vi "ST_do_SQL_transaction.vi"(6 "station":T1, 8 "error_in":errorcluster, 10 "SQL_transaction":string[](array[string]), 11 "SQL_connection_reference":T2) -> (0 "error_out":errorcluster)   [LabVIEW 2020]
uses:
  <vilib>/addons/database/Connection.llb/Conn ObjectReference.ctl
  station.ctl
  <vilib>/addons/database/Auxilliary.llb/DB Tools Transaction.ctl
  FGV/DIAGNOSTICS_message_history_buffer/FGV_PROXY_DIAGNOSTICS_message_history_buffer.ctl
  <vilib>/addons/database/Connection.llb/Conn Transaction.vi
  <vilib>/addons/database/Connection.llb/Conn Execute.vi
  <vilib>/addons/database/Recordset.llb/Rec Destroy - Connection.vi
  <vilib>/addons/database/NI_Database_API.lvlib
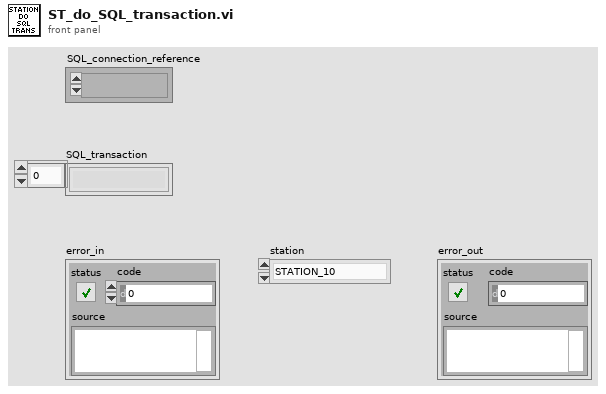
[diagram p1: front panel]
types:
  T1 = typedef "station.ctl" = enum16{"STATION_10", "STATION_20", "STATION_30", "STATION_40", "STATION_50", "STATION_60", "STATION_70", "STATION_80", "STATION_90", "STATION_100", "STATION_110", "STATION_120", "STATION_165", "MAIN"}
  T2 = typedef "NI_Database_API.lvlib/Conn ObjectReference.ctl" = refnum<k1>
  T3 = typedef "FGV_PROXY_DIAGNOSTICS_message_history_buffer.ctl" = enum16{"initialize", "add_TCP_PLC_to_PC", "add_TCP_PC_to_PLC", "add_SQL_PC_to_DB", "add_SQL_transaction", "add_SQL_DB_to_PC", "get_station", "get_all", "clear_station", "clear_all", "save_log"}
  T4 = typedef "NI_Database_API.lvlib/DB Tools Transaction.ctl" = enum16{"begin", "commit", "rollback"}
  T5 = typedef "NI_Database_API.lvlib/Rec ObjectReference.ctl" = refnum<k1>
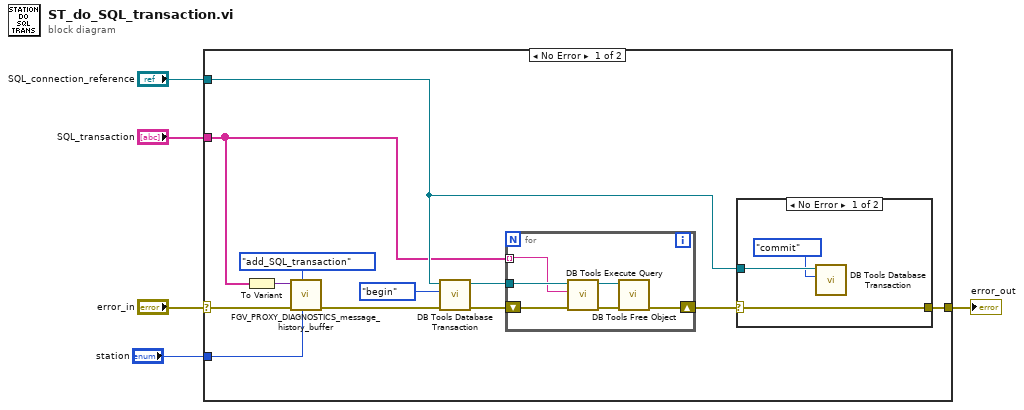
[diagram p0: block diagram]
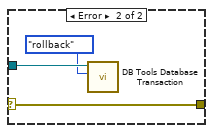
[diagram p2: hidden frame]
diagram:
  n1 = case shown="No Error" "error_in" {
    selector: "error_in" -> [w9 w30]
    tunnel: [w13 w30] -> w5
    tunnel: "SQL_transaction" -> [w7 _]
    tunnel: "SQL_connection_reference" -> [w12 _]
    tunnel: "station" -> [w6 _]
    frame No Error {
      n2 = To Variant(anything=w7) -> (Variant=w11:variant)
      n3 = call "FGV_PROXY_DIAGNOSTICS_message_history_buffer.vi"("station"=w6, "options"=FGV_PROXY_DIAGNOSTICS_message_history_buffer."add_SQL_transaction", "error_in"=w9, "input"=w11) -> ("error_out"=w8:errorcluster)  [unwired: 6 in, 1 out]
      n4 = call-poly <vilib>:"DB Tools Database Transaction.vi"("error in (no error)"=w8, "operation (begin)"=DB_Tools_Transaction."begin", "connection reference"=w12) -> ("error out"=w16:errorcluster, "connection reference out"=w15:T2)  [unwired: 3 in]
      n5 = for {
        tunnel: w15 -> [w20]
        shift-right: [w19] -> w14
        shift-left: w16 -> [w21]
        tunnel: w7 -> [w18] mode=indexing
        n6 = call-poly <vilib>:"DB Tools Execute Query.vi"("error in (no error)"=w21, "SQL query"=w18, "connection reference"=w20) -> ("error out"=w22:errorcluster, "recordset reference"=w23:T5)  [unwired: 5 in]
        n7 = call-poly <vilib>:"DB Tools Free Object.vi"("error in (no error)"=w22, "recordset reference"=w23) -> ("error out"=w19:errorcluster)  [unwired: 8 in, 1 out]
      }
      n8 = case shown="No Error" w14 {
        selector: w14 -> [w24 w27]
        tunnel: w12 -> [w26 w29]
        tunnel: [w24 w27] -> w13
        frame No Error {
          n9 = call-poly <vilib>:"DB Tools Database Transaction.vi"("operation (begin)"=DB_Tools_Transaction."commit", "connection reference"=w26) -> ()  [unwired: 4 in, 2 out]
        }
        frame Error {
          n10 = call-poly <vilib>:"DB Tools Database Transaction.vi"("operation (begin)"=DB_Tools_Transaction."rollback", "connection reference"=w29) -> ()  [unwired: 4 in, 2 out]
        }
      }
    }
    frame Error {
    }
  }
  "error_out" <- w5
